vi "Close.vi"(8 "error in (no error)":errorcluster, 11 "Parallax Standard Servo in":refnum<class "Parallax Standard Servo.lvclass">) -> (0 "error out":errorcluster)   [LabVIEW 2019, in "Parallax Standard Servo.lvclass"]
doc: "Terminates the software connection to the sensor."
uses:
  Parallax Standard Servo.lvclass
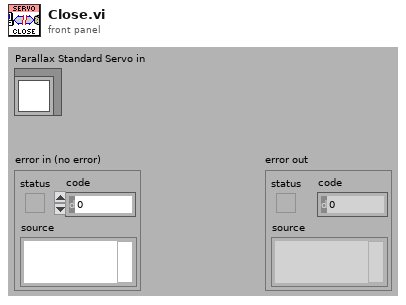
[diagram p1: front panel]
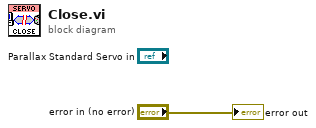
[diagram p0: block diagram]
diagram:
  "error out" <- "error in (no error)"
